vi "sterowanieRobot.vi"() -> ()   [LabVIEW 2017]
doc: "The myRIO Project template acquires acceleration data from the onboard accelerometer and displays the changes of acceleration values in a waveform chart."
uses:
  <vilib>/myRIO/Instrument Drivers/Onboard IO/DIO/typedefs/DIO Reference.ctl
  <vilib>/myRIO/Common/Instrument Driver Framework/Utilities/typedefs/myRIO Generic Hardware Reference.ctl
  <vilib>/myRIO/Common/Instrument Driver Framework/Utilities/typedefs/Hardware Version Enum.ctl
  <vilib>/myRIO/Common/Instrument Driver Framework/Utilities/typedefs/myRIO v1.0 Reference.ctl
  <vilib>/myRIO/Common/Instrument Driver Framework/Utilities/typedefs/Generic FPGA Reference.ctl
  <vilib>/myRIO/Common/Instrument Driver Framework/myRIO v1.0/DIO/typedefs/DIO Channels List.ctl
  <vilib>/myRIO/Common/Instrument Driver Framework/myRIO v1.0/DIO/typedefs/DIO Channels Enum.ctl
  <vilib>/userdefined/High Color/nirio_resource_hc.ctl
  <vilib>/myRIO/Instrument Drivers/Onboard IO/UART/typedef/VISA Configuration.ctl
  <vilib>/myRIO/Instrument Drivers/Onboard IO/PWM/typedefs/PWM Reference.ctl
  <vilib>/myRIO/Common/Instrument Driver Framework/myRIO v1.0/PWM/typedefs/PWM Channels Enum.ctl
  <vilib>/myRIO/Instrument Drivers/Onboard IO/PWM/typedefs/PWM Configuration.ctl
  <vilib>/myRIO/Common/Instrument Driver Framework/Utilities/vis/Is FPGA Ref Available.vi
  <vilib>/myRIO/Common/Instrument Driver Framework/myRIO v1.0/DIO/vis/myRIO v1.1 Open DIO.vi
  <vilib>/myRIO/Instrument Drivers/Onboard IO/DIO/vis/Write.vi
  <vilib>/myRIO/Common/Instrument Driver Framework/myRIO v1.0/PWM/vis/myRIO v1.1 Open PWM.vi
  <vilib>/myRIO/Instrument Drivers/Onboard IO/PWM/vis/Set Duty Cycle and Frequency.vi
  <vilib>/myRIO/Common/Instrument Driver Framework/Utilities/vis/Validate Channels.vi
  <vilib>/myRIO/Common/Instrument Driver Framework/myRIO v1.0/DIO/vis/myRIO v1.0 Reserve DIO.vi
  <vilib>/myRIO/Common/Instrument Driver Framework/myRIO v1.0/PWM/vis/myRIO v1.0 Reserve PWM.vi
  <vilib>/myRIO/Common/Instrument Driver Framework/myRIO v1.0/Resource Manager/vis/myRIO v1.0 Reserve Channel List.vi
  <vilib>/myRIO/Common/Instrument Driver Framework/myRIO v1.0/DIO/vis/myRIO v1.0 Build MUX Configuration DIO.vi
  <vilib>/myRIO/Common/Instrument Driver Framework/myRIO v1.0/PWM/vis/myRIO v1.0 Build MUX Configuration PWM.vi
  <vilib>/myRIO/Common/Instrument Driver Framework/myRIO v1.0/Resource Manager/vis/myRIO v1.0 Reserve Channel.vi
  <vilib>/myRIO/Common/Instrument Driver Framework/myRIO v1.0/Resource Manager/vis/myRIO v1.0 Unreserve Channel.vi
  <vilib>/myRIO/Common/Instrument Driver Framework/myRIO v1.0/Resource Manager/vis/myRIO v1.0 Create Configuration List.vi
  <vilib>/myRIO/Common/Instrument Driver Framework/myRIO v1.0/Resource Manager/vis/myRIO v1.0 Build Mutex Name.vi
  <vilib>/Utility/VariantDataType/GetNumericInfo.vi
  <vilib>/Utility/error.llb/Error Cluster From Error Code.vi
  <vilib>/myRIO/Common/Instrument Driver Framework/myRIO v1.0/myRIO v1.1 Open.vi
  <vilib>/myRIO/Common/Instrument Driver Framework/Utilities/vis/IO Manager.vi
  <vilib>/myRIO/Common/Instrument Driver Framework/Utilities/vis/Configuration Manager.vi
  <vilib>/myRIO/Common/Instrument Driver Framework/myRIO v1.0/Resource Manager/vis/myRIO v1.0 Configure IO.vi
  <vilib>/myRIO/Common/Instrument Driver Framework/myRIO v1.0/myRIO v1.0 Close.vi
  <vilib>/myRIO/Common/Instrument Driver Framework/myRIO v1.0/PWM/vis/myRIO v1.0 Write PWM.vi
  <vilib>/myRIO/Common/Instrument Driver Framework/myRIO v1.0/DIO/vis/myRIO v1.0 Write DIO.vi
  <vilib>/Instr/_visa.llb/VISA Configure Serial Port (Instr).vi
  <vilib>/myRIO/Express VI/Onboard IO/PWM/PWM Express VI.xnode
  <vilib>/myRIO/Instrument Drivers/Onboard IO/PWM/vis/myRIO PWM Open.xnode
  <vilib>/myRIO/Express VI/Onboard Devices/LED/LED Express VI.xnode
  <vilib>/myRIO/Instrument Drivers/Onboard IO/DIO/vis/myRIO DIO Open.xnode
  <vilib>/myRIO/Express VI/Onboard IO/UART/UART Express VI.xnode
  <vilib>/myRIO/Instrument Drivers/Onboard IO/PWM/PWM.lvlib
  <vilib>/myRIO/Instrument Drivers/Onboard IO/DIO/DIO.lvlib
  <vilib>/myRIO/Instrument Drivers/Onboard IO/UART/UART.lvlib
panel:
  out "SP":dbl
  out "S1":dbl
  out "S2":dbl
  out "S3":dbl
  out "S4":dbl
  out "Sn":dbl
  out "StringPlatforma":string
  out "Napięcie akumulatorów":dbl
  out "Temperatura":dbl
  out "Położenie osi skrętnej":u16(knob) scale=0.0..99.0
  out "Zabezpieczenie wyłączenie PWM":string
  out "Kierunek skrętu(1-prawo, 2-lewo)":string
  out "Kierunek jazdy(0-postój, 1-do przodu, 2-do tyłu)":string
  out "Characters Read":string
  in  "Wi-Fi test":bool
  out "duty cycleSP [%]":dbl
  out "pulse widthSP [ms]":dbl=1.5
  out "duty cycleS1b [%]":dbl
  out "pulse widthS1b [ms]":dbl=1.5
  out "duty cycleS1a [%]":dbl
  out "pulse widthS1a [ms]":dbl=1.5
  out "duty cycleS2 [%]":dbl
  out "pulse widthS2 [ms]":dbl=1.5
  out "duty cycleS3 [%]":dbl
  out "pulse widthS3 [ms]":dbl=1.5
  out "duty cycleS4 [%]":dbl
  out "pulse widthS4 [ms]":dbl=1.5
  in  "[STOP]":bool
  out "pulse widthSn [ms]":dbl=1.5
  out "duty cycleSn [%]":dbl
  # "Sterowanie Manipulator"
  # "T - ręczne\nF - rękawica"
  # "Sterowanie Podstawa"
  # "Informacje zwrotne platforma"
  # "Informacje zwrotne rękawica"
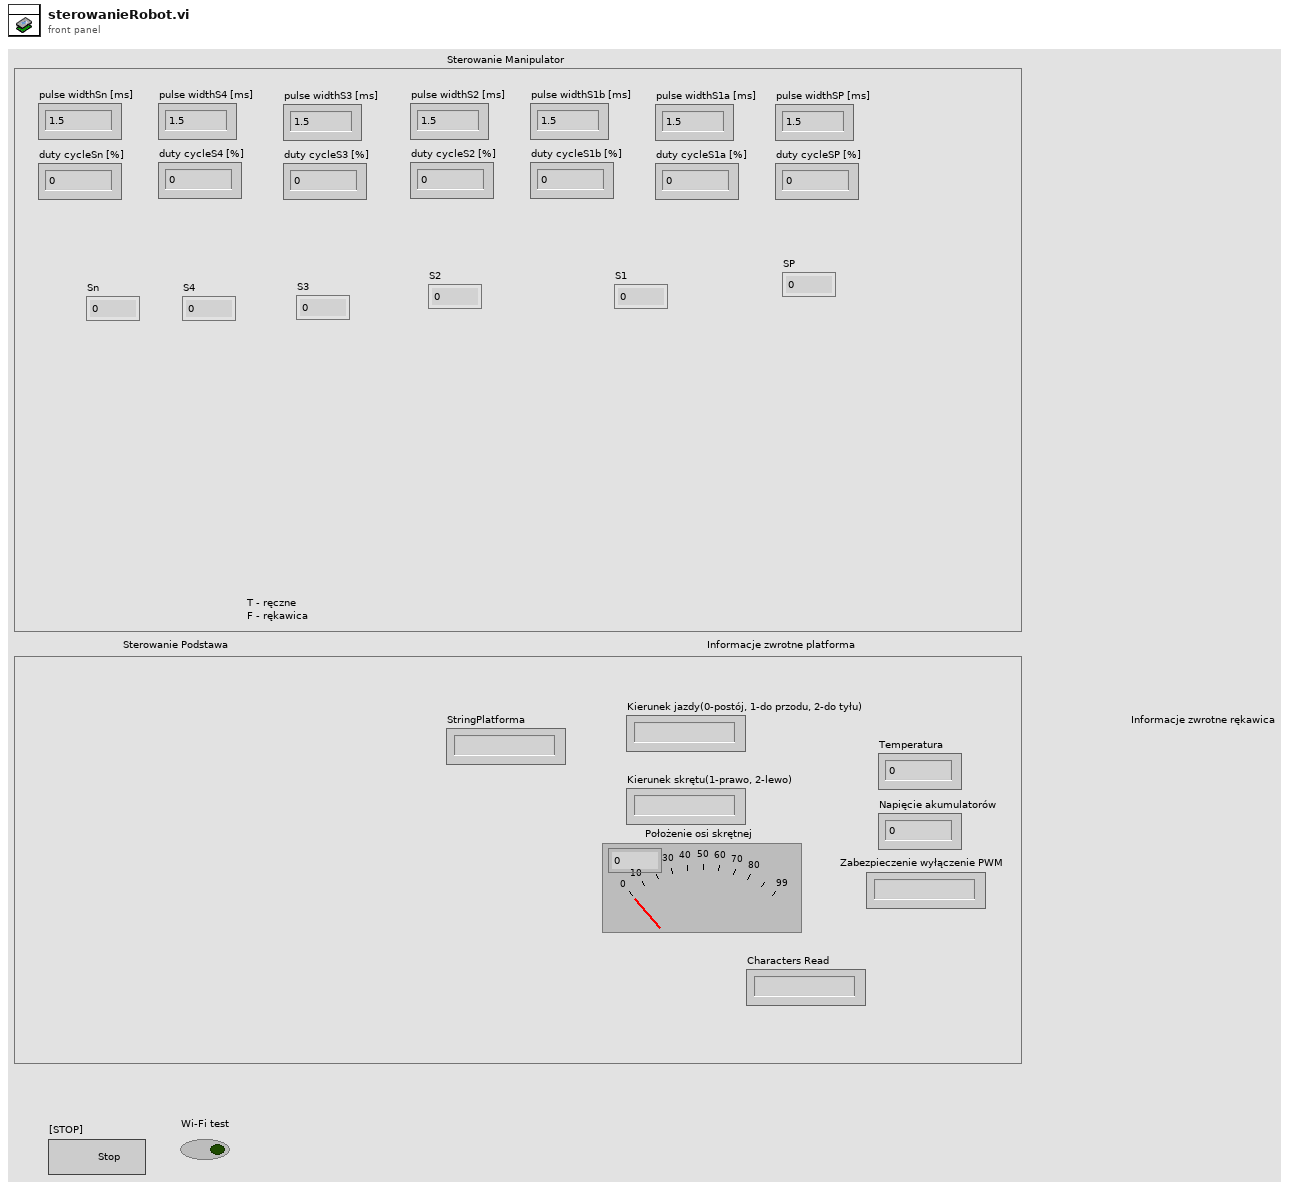
[diagram p1: front panel]
types:
  T1 = typedef "PWM.lvlib/PWM Reference.ctl" = cluster{"myRIO Reference":T2, "PWM Channels Enum":T6, "PWM Configuration":T7}
  T2 = typedef "myRIO Generic Hardware Reference.ctl" = cluster{"myRIO Model":T3, "myRIO Hardware Reference":T4}
  T3 = typedef "Hardware Version Enum.ctl" = enum16{"Unknown", "myRIO-1900", "myRIO-1950", "roboRIO", "NI ELVIS RIO CM"}
  T4 = typedef "myRIO v1.0 Reference.ctl" = cluster{"Generic FPGA Reference":T5, "Allow multiple opens":bool}
  T5 = typedef "Generic FPGA Reference.ctl" = refnum<k20>
  T6 = typedef "PWM Channels Enum.ctl" = enum16{"Not Connected", "C/PWM0", "C/PWM1", "A/PWM0", "A/PWM1", "A/PWM2", "B/PWM0", "B/PWM1", "B/PWM2", "PWM/PWM0", "PWM/PWM1", "PWM/PWM2", "PWM/PWM3", "PWM/PWM4", "PWM/PWM5", "PWM/PWM6", "PWM/PWM7", "PWM/PWM8", "PWM/PWM9"}
  T7 = typedef "PWM.lvlib/PWM Configuration.ctl" = cluster{"Frequency":dbl, "Duty Cycle":dbl}
  T8 = typedef "nirio_resource_hc.ctl" = tag
  T9 = typedef "DIO.lvlib/DIO Reference.ctl" = cluster{"myRIO Reference":T2, "DIO Channels List":T10}
  T10 = typedef "DIO Channels List.ctl" = T11[]
  T11 = typedef "DIO Channels Enum.ctl" = enum16{"Not Connected", "C/DIO0", "C/DIO1", "C/DIO2", "C/DIO3", "C/DIO4", "C/DIO5", "C/DIO6", "C/DIO7", "A/DIO0", "A/DIO1", "A/DIO2", "A/DIO3", "A/DIO4", "A/DIO5", "A/DIO6", "A/DIO7", "A/DIO8", "A/DIO9", "A/DIO10", "A/DIO11", "A/DIO12", "A/DIO13", "A/DIO14", "A/DIO15", "B/DIO0", "B/DIO1", "B/DIO2", "B/DIO3", "B/DIO4", "B/DIO5", "B/DIO6", "B/DIO7", "B/DIO8", "B/DIO9", "B/DIO10", "B/DIO11", "B/DIO12", "B/DIO13", "B/DIO14", "B/DIO15", "LED0", "LED1", "LED2", "LED3", "Button0", "DIO/DIO0", "DIO/DIO1", "DIO/DIO2", "DIO/DIO3", "DIO/DIO4", "DIO/DIO5", "DIO/DIO6", "DIO/DIO7", "DIO/DIO8", "DIO/DIO9", "SPI/CS0", "SPI/CS1", "SPI/CS2", "SPI/CS3", "LED RADIO (Green)", "LED RADIO (Red)", "LED COMM (Green)", "LED COMM (Red)", "LED MODE (Green)", "LED MODE (Red)"}
  T12 = typedef "UART.lvlib/VISA Configuration.ctl" = cluster{"baud rate (9600)":u32, "data bits (8)":u16, "parity (0:none)":enum16{"None", "Odd", "Even", "Mark", "Space"}, "stop bits (10: 1 bit)":u16, "flow control (0:none)":u16, "termination char\n(0xA = '\\n' = LF) ":u8, "Enable Termination\nChar (T)":bool, "timeout (10sec)":u32}
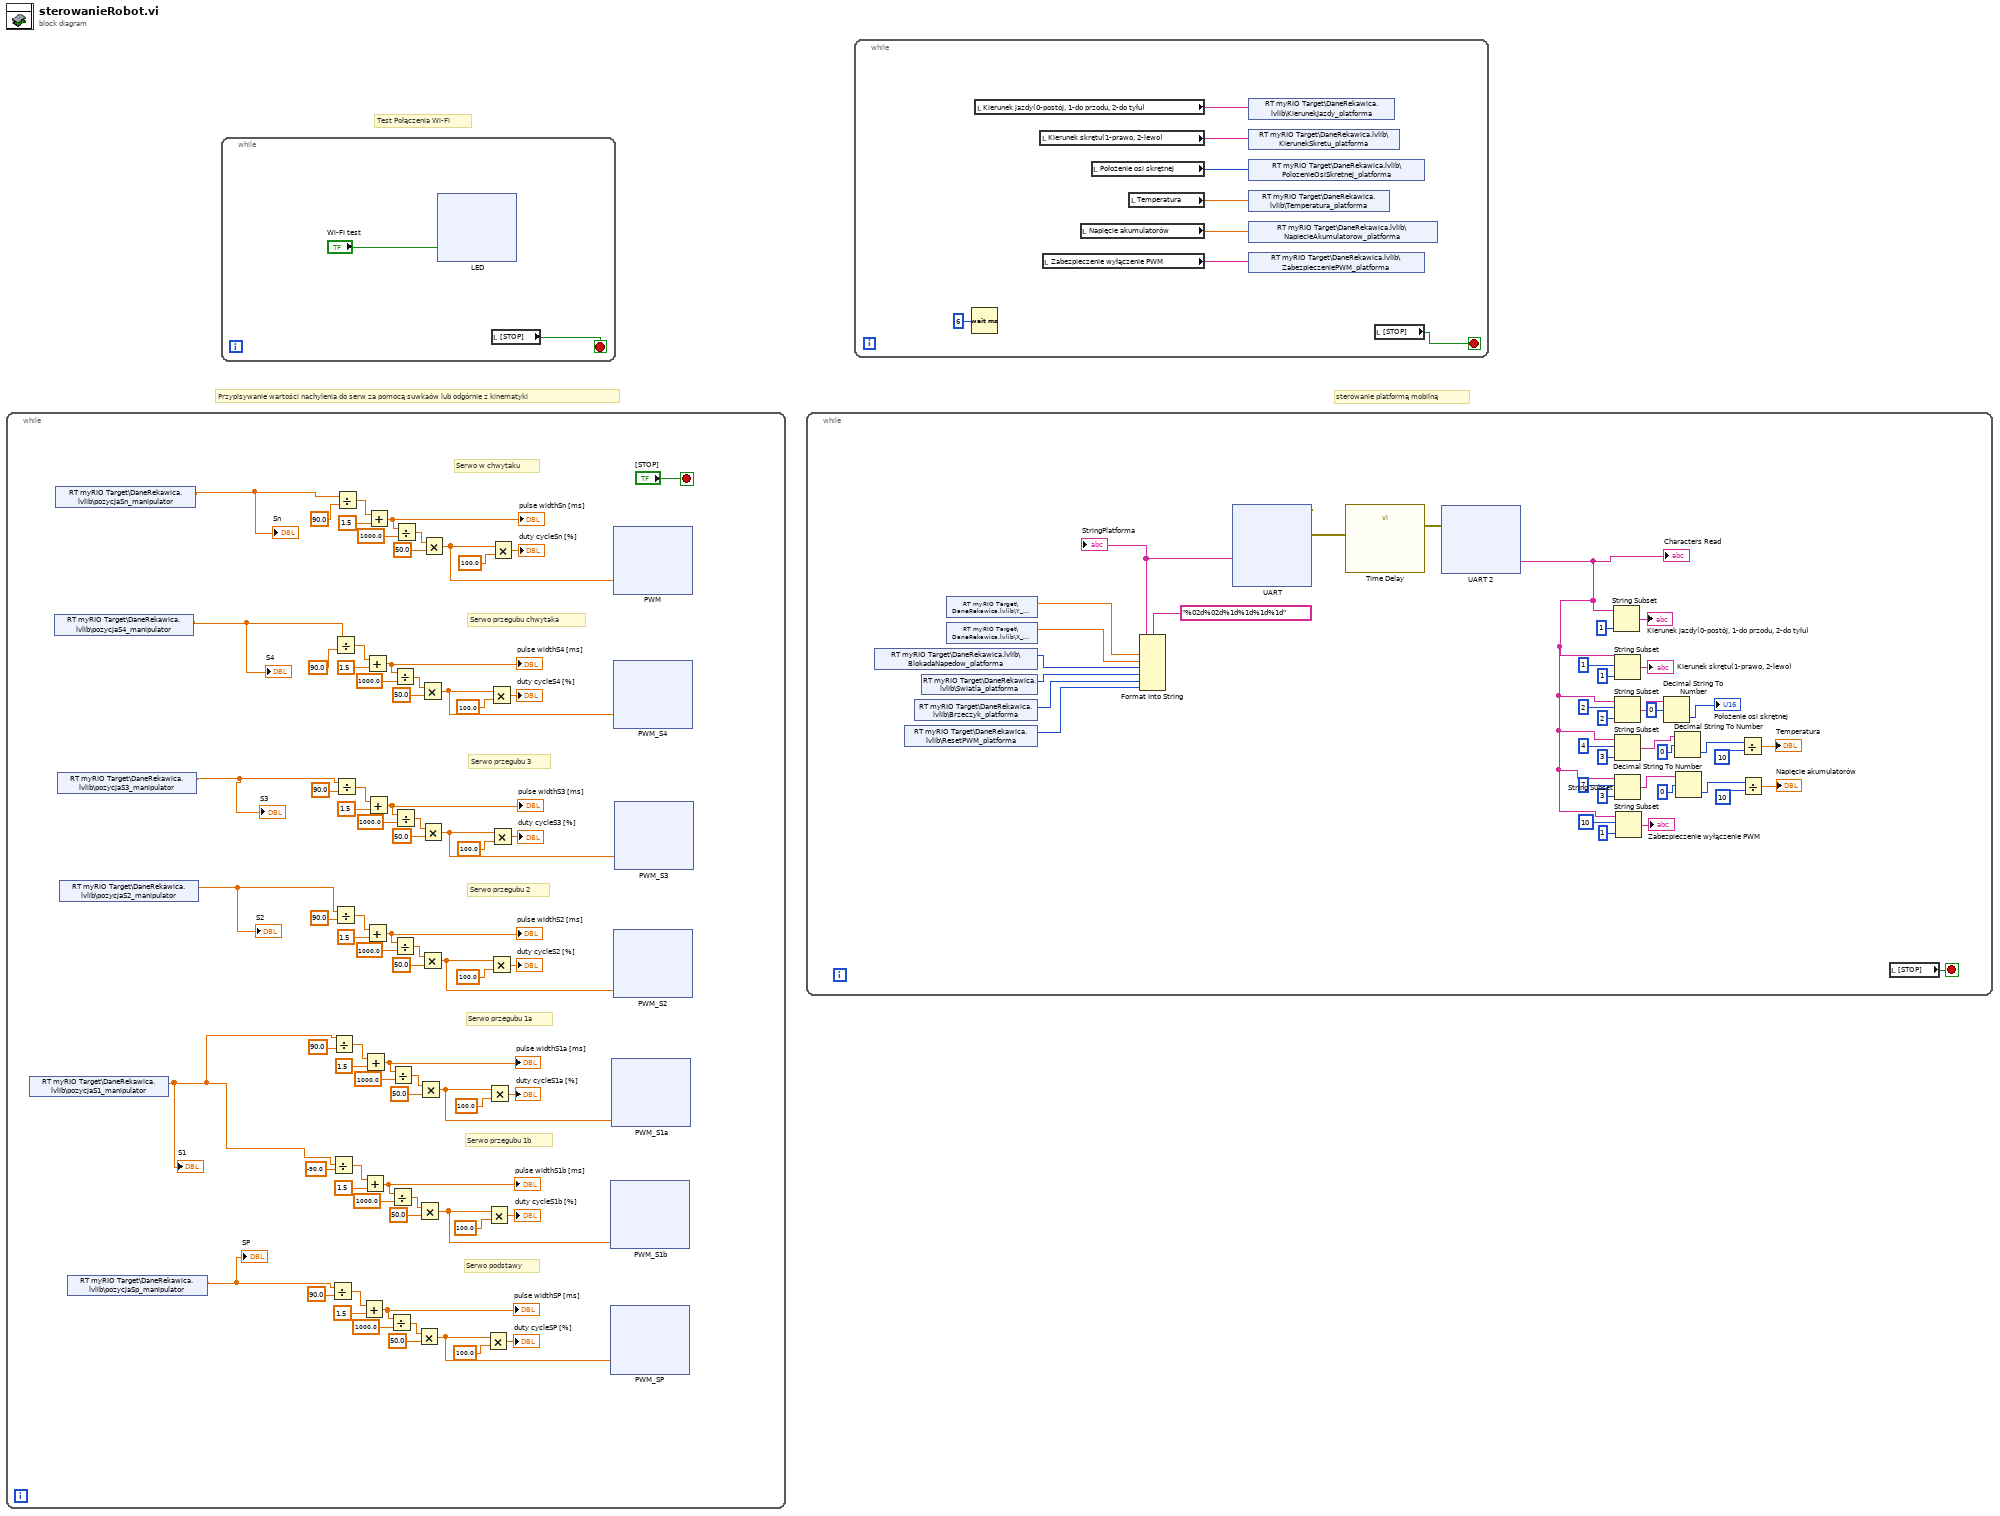
[diagram p0: block diagram]
diagram:
  # "sterowanie platformą mobilną"
  # "Test Połączenia Wi-Fi"
  # "Przypisywanie wartości nachylenia do serw za pomocą suwkaów lub odgórnie z kinematyki"
  n1 = while {
    stop <- "[STOP]" stop-if-true
    # "Serwo podstawy"
    # "Serwo przegubu 1b"
    # "Serwo przegubu 1a"
    # "Serwo przegubu 2"
    # "Serwo przegubu 3"
    # "Serwo przegubu chwytaka"
    # "Serwo w chwytaku"
    n2 = shared-variable "RT myRIO Target\\DaneRekawica.lvlib\\pozycjaS1_manipulator"() -> (w2:dbl)  [unwired: 1 in, 1 out]
    "S1" <- w2
    n3 = shared-variable "RT myRIO Target\\DaneRekawica.lvlib\\pozycjaS4_manipulator"() -> (w5:dbl)  [unwired: 1 in, 1 out]
    "S4" <- w5
    n4 = shared-variable "RT myRIO Target\\DaneRekawica.lvlib\\pozycjaSn_manipulator"() -> (w6:dbl)  [unwired: 1 in, 1 out]
    "Sn" <- w6
    n5 = shared-variable "RT myRIO Target\\DaneRekawica.lvlib\\pozycjaS3_manipulator"() -> (w4:dbl)  [unwired: 1 in, 1 out]
    "S3" <- w4
    n6 = shared-variable "RT myRIO Target\\DaneRekawica.lvlib\\pozycjaS2_manipulator"() -> (w3:dbl)  [unwired: 1 in, 1 out]
    "S2" <- w3
    n7 = shared-variable "RT myRIO Target\\DaneRekawica.lvlib\\pozycjaSp_manipulator"() -> (w1:dbl)  [unwired: 1 in, 1 out]
    "SP" <- w1
    n8 = Divide(x=w1, y=90.0) -> (x/y=w15:dbl)
    n9 = Divide(x=w2, y=-90.0) -> (x/y=w25:dbl)
    n10 = Divide(x=w2, y=90.0) -> (x/y=w35:dbl)
    n11 = Divide(x=w5, y=90.0) -> (x/y=w65:dbl)
    n12 = Divide(x=w3, y=90.0) -> (x/y=w45:dbl)
    n13 = Divide(x=w4, y=90.0) -> (x/y=w55:dbl)
    n14 = Divide(x=w6, y=90.0) -> (x/y=w76:dbl)
    n15 = Add(x=w15, y=1.5) -> (x+y=w13:dbl)
    "pulse widthSP [ms]" <- w13
    n16 = Add(x=w25, y=1.5) -> (x+y=w23:dbl)
    "pulse widthS1b [ms]" <- w23
    n17 = Add(x=w35, y=1.5) -> (x+y=w33:dbl)
    "pulse widthS1a [ms]" <- w33
    n18 = Add(x=w65, y=1.5) -> (x+y=w63:dbl)
    "pulse widthS4 [ms]" <- w63
    n19 = Add(x=w45, y=1.5) -> (x+y=w43:dbl)
    "pulse widthS2 [ms]" <- w43
    n20 = Add(x=w55, y=1.5) -> (x+y=w53:dbl)
    "pulse widthS3 [ms]" <- w53
    n21 = Add(x=w76, y=1.5) -> (x+y=w74:dbl)
    "pulse widthSn [ms]" <- w74
    n22 = Divide(x=w13, y=1000.0) -> (x/y=w11:dbl)
    n23 = Divide(x=w23, y=1000.0) -> (x/y=w21:dbl)
    n24 = Divide(x=w33, y=1000.0) -> (x/y=w31:dbl)
    n25 = Divide(x=w63, y=1000.0) -> (x/y=w61:dbl)
    n26 = Divide(x=w43, y=1000.0) -> (x/y=w41:dbl)
    n27 = Divide(x=w53, y=1000.0) -> (x/y=w51:dbl)
    n28 = Divide(x=w74, y=1000.0) -> (x/y=w72:dbl)
    n29 = Multiply(x=w11, y=50.0) -> (x*y=w8:dbl)
    n30 = Multiply(x=w21, y=50.0) -> (x*y=w18:dbl)
    n31 = Multiply(x=w31, y=50.0) -> (x*y=w28:dbl)
    n32 = Multiply(x=w61, y=50.0) -> (x*y=w58:dbl)
    n33 = Multiply(x=w41, y=50.0) -> (x*y=w38:dbl)
    n34 = Multiply(x=w51, y=50.0) -> (x*y=w48:dbl)
    n35 = Multiply(x=w72, y=50.0) -> (x*y=w69:dbl)
    n36 = Multiply(x=w8, y=100.0) -> (x*y=→"duty cycleSP [%]":dbl)
    n37 = Multiply(x=w18, y=100.0) -> (x*y=→"duty cycleS1b [%]":dbl)
    n38 = Multiply(x=w28, y=100.0) -> (x*y=→"duty cycleS1a [%]":dbl)
    n39 = Multiply(x=w58, y=100.0) -> (x*y=→"duty cycleS4 [%]":dbl)
    n40 = Multiply(x=w38, y=100.0) -> (x*y=→"duty cycleS2 [%]":dbl)
    n41 = Multiply(x=w48, y=100.0) -> (x*y=→"duty cycleS3 [%]":dbl)
    n42 = Multiply(x=w69, y=100.0) -> (x*y=→"duty cycleSn [%]":dbl)
    n43 = xnode "PWM_SP"("Duty Cycle"=w8) -> ()  [unwired: 1 in, 1 out]
    n44 = xnode "PWM_S1b"("Duty Cycle"=w18) -> ()  [unwired: 1 in, 1 out]
    n45 = xnode "PWM_S1a"("Duty Cycle"=w28) -> ()  [unwired: 1 in, 1 out]
    n46 = xnode "PWM"("Duty Cycle"=w69) -> ()  [unwired: 1 in, 1 out]
    n47 = xnode "PWM_S4"("Duty Cycle"=w58) -> ()  [unwired: 1 in, 1 out]
    n48 = xnode "PWM_S2"("Duty Cycle"=w38) -> ()  [unwired: 1 in, 1 out]
    n49 = xnode "PWM_S3"("Duty Cycle"=w48) -> ()  [unwired: 1 in, 1 out]
  }
  n50 = while {
    stop <- w323 stop-if-true
    n51 = xnode "LED"("wi-fi"="Wi-Fi test") -> ()  [unwired: 1 in, 1 out]
    n52 = local read "[STOP]"() -> (w323:bool)
  }
  n53 = while {
    stop <- w398 stop-if-true
    n54 = shared-variable "RT myRIO Target\\DaneRekawica.lvlib\\BlokadaNapedow_platforma"() -> (w363:i8)  [unwired: 1 in, 1 out]
    n55 = shared-variable "RT myRIO Target\\DaneRekawica.lvlib\\ResetPWM_platforma"() -> (w360:i8)  [unwired: 1 in, 1 out]
    n56 = shared-variable "RT myRIO Target\\DaneRekawica.lvlib\\Brzeczyk_platforma"() -> (w361:i8)  [unwired: 1 in, 1 out]
    n57 = shared-variable "RT myRIO Target\\DaneRekawica.lvlib\\Swiatla_platforma"() -> (w362:i8)  [unwired: 1 in, 1 out]
    n58 = shared-variable "RT myRIO Target\\DaneRekawica.lvlib\\Y_platforma"() -> (w365:dbl)  [unwired: 1 in, 1 out]
    n59 = shared-variable "RT myRIO Target\\DaneRekawica.lvlib\\X_platforma"() -> (w364:dbl)  [unwired: 1 in, 1 out]
    n60 = Format Into String(format string="%02d%02d%1d%1d%1d%1d", w365, w364, w363, w362, w361, w360) -> (resulting string=w369:string)  [unwired: 2 in, 1 out]
    "StringPlatforma" <- w369
    n61 = xnode "UART"("Characters to Write"=w369) -> ("error out"=w367:errorcluster)  [unwired: 1 in, 1 out]
    n62 = call "Time Delay"("error in (no error)"=w367) -> ("error out"=w366:errorcluster)  [unwired: 10 in]
    n63 = xnode "UART 2"("error in (no error)"=w366) -> ("Characters Read"=w370:string)  [unwired: 1 out]
    "Characters Read" <- w370
    n64 = String Subset(string=w370, length (rest)=1 ("length (rest)")) -> (substring=→"Kierunek jazdy(0-postój, 1-do przodu, 2-do tyłu)":string)  [unwired: 1 in]
    n65 = String Subset(string=w370, offset (0)=1, length (rest)=1 ("length (rest)")) -> (substring=→"Kierunek skrętu(1-prawo, 2-lewo)":string)
    n66 = String Subset(string=w370, offset (0)=2, length (rest)=2 ("length (rest)")) -> (substring=w383:string)
    n67 = String Subset(string=w370, offset (0)=4, length (rest)=3 ("length (rest)")) -> (substring=w379:string)
    n68 = String Subset(string=w370, offset (0)=7, length (rest)=3 ("length (rest)")) -> (substring=w371:string)
    n69 = String Subset(string=w370, offset (0)=10, length (rest)=1 ("length (rest)")) -> (substring=→"Zabezpieczenie wyłączenie PWM":string)
    n70 = Decimal String To Number(string=w383, offset=0) -> (number=→"Położenie osi skrętnej":i32)  [unwired: 1 in, 1 out]
    n71 = Decimal String To Number(string=w379, offset=0) -> (number=w378:i32)  [unwired: 1 in, 1 out]
    n72 = Decimal String To Number(string=w371, offset=0) -> (number=w374:i32)  [unwired: 1 in, 1 out]
    n73 = Divide(x=w378, y=10) -> (x/y=→"Temperatura":dbl)
    n74 = Divide(x=w374, y=10) -> (x/y=→"Napięcie akumulatorów":dbl)
    n75 = local read "[STOP]"() -> (w398:bool)
  }
  n76 = while {
    stop <- w439 stop-if-true
    n77 = Wait (ms)(milliseconds to wait=u32 6) -> ()  [unwired: 1 out]
    n78 = local read "Kierunek jazdy(0-postój, 1-do przodu, 2-do tyłu)"() -> (w438:string)
    n79 = local read "Kierunek skrętu(1-prawo, 2-lewo)"() -> (w437:string)
    n80 = local read "Zabezpieczenie wyłączenie PWM"() -> (w433:string)
    n81 = local read "Napięcie akumulatorów"() -> (w434:dbl)
    n82 = local read "Położenie osi skrętnej"() -> (w436:u16)
    n83 = local read "Temperatura"() -> (w435:dbl)
    n84 = shared-variable "RT myRIO Target\\DaneRekawica.lvlib\\KierunekJazdy_platforma"(w438) -> ()  [unwired: 1 in, 1 out]
    n85 = shared-variable "RT myRIO Target\\DaneRekawica.lvlib\\KierunekSkretu_platforma"(w437) -> ()  [unwired: 1 in, 1 out]
    n86 = shared-variable "RT myRIO Target\\DaneRekawica.lvlib\\PolozenieOsiSkretnej_platforma"(w436) -> ()  [unwired: 1 in, 1 out]
    n87 = shared-variable "RT myRIO Target\\DaneRekawica.lvlib\\Temperatura_platforma"(w435) -> ()  [unwired: 1 in, 1 out]
    n88 = shared-variable "RT myRIO Target\\DaneRekawica.lvlib\\NapiecieAkumulatorow_platforma"(w434) -> ()  [unwired: 1 in, 1 out]
    n89 = shared-variable "RT myRIO Target\\DaneRekawica.lvlib\\ZabezpieczeniePWM_platforma"(w433) -> ()  [unwired: 1 in, 1 out]
    n90 = local read "[STOP]"() -> (w439:bool)
  }
